vi "Create Task.vi"(8 "error in (no error)":errorcluster, 9 "Task Type":string, 10 "Task Name":string, 11 "Node in":refnum<class "Node.lvclass">) -> (0 "error out":errorcluster, 2 "Task":refnum<class "Task.lvclass">, 3 "Node out":refnum<class "Node.lvclass">)   [LabVIEW 2020, in "VolatusConfig.lvlib" / "Node.lvclass"]
uses:
  Node.lvclass
  Node.lvclass/Node.ctl
  VolatusConfigElement/VolatusConfigElement.lvclass
  VolatusConfig.lvlib
  Meta Type.ctl
  lv-cdm/CDM-Config/Config Filter/Config Lookup.lvclass
  C:/dev/lv20CE/relink/lv-volatus/VolatusConfig/VolatusConfigElement/VolatusConfigElement.lvclass
  C:/dev/lv20CE/relink/lv-volatus/VolatusConfig/Node/Node.lvclass
  Task/Task.lvclass
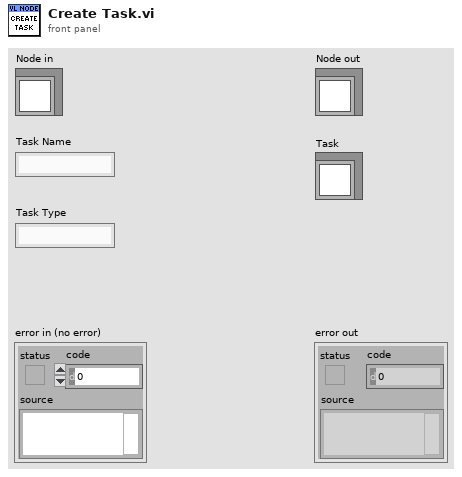
[diagram p1: front panel]
types:
  T1 = typedef "VolatusConfig.lvlib/Meta Type.ctl" = enum16{"UNKNOWN", "VL_System", "VL_Cluster", "VL_Node", "VL_Task", "VL_Group", "VL_Channel", "VL_Task_List", "VL_Scaling", "VL_Sensor", "VL_Sensor_List", "VL_Scale"}
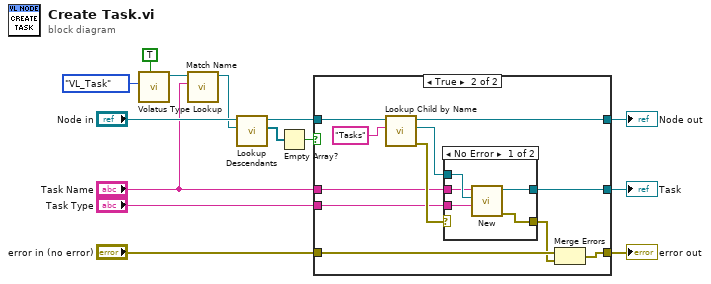
[diagram p0: block diagram]
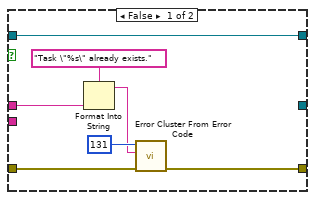
[diagram p2: hidden frame]
diagram:
  n1 = call "Volatus Type Lookup.vi"("Don't Recurse Past Match (F)"=TRUE, "Meta Type"=Meta_Type."VL_Task") -> ("Config Lookup out"=w12:refnum<class "Config Lookup.lvclass">)  [unwired: 8 in, 1 out]
  n2 = call "Match Name.vi"("Name"="Task Name", "Config Lookup (New)"=w12) -> ("Config Lookup out"=w11:refnum<class "Config Lookup.lvclass">)  [unwired: 8 in, 1 out]
  n3 = call "Lookup Descendants.vi"("Lookup"=w11, "VolatusConfigElement in"="Node in") -> ("Descendants"=w9:refnum<class "Config Element.lvclass">[], "VolatusConfigElement out"=w8:refnum<class "Node.lvclass">)  [unwired: 7 in, 1 out]
  n4 = Empty Array?(array=w9) -> (empty?=w7:bool)
  n5 = case shown="True" w7 {
    tunnel: w8 -> [w15 w32]
    tunnel: "error in (no error)" -> [w21 w26]
    tunnel: "Task Name" -> [w19 w28]
    tunnel: "Task Type" -> [_ w27]
    tunnel: [w16 w24] -> w3
    tunnel: [_ w23] -> w2
    tunnel: [w15 w22] -> w1
    frame False {
      n6 = Format Into String(format string="Task \"%s\" already exists.", w19) -> (resulting string=w17:string)  [unwired: 2 in, 1 out]
      n7 = call <vilib>:"Error Cluster From Error Code.vi"("error in (no error)"=w21, "error message (\"\")"=w17, "error code (0)"=131) -> ("error out"=w16:errorcluster)  [unwired: 6 in]
    }
    frame True {
      n8 = call "Lookup Child by Name.vi"("Child Name"="Tasks", "VolatusConfigElement in"=w32) -> ("error out"=w29:errorcluster, "Child"=w30:refnum<class "Config Element.lvclass">, "VolatusConfigElement out"=w22:refnum<class "Node.lvclass">)  [unwired: 6 in, 1 out]
      n9 = case shown="No Error" w29 {
        selector: w29 -> [_ w38]
        tunnel: w30 -> [w37 _]
        tunnel: w28 -> [w36 _]
        tunnel: [w34 w38] -> w25
        tunnel: w27 -> [w35 _]
        tunnel: [w33 _] -> w23
        frame No Error {
          n10 = call "New.vi"("Type"=w35, "Parent"=w37, "Name"=w36) -> ("error out"=w34:errorcluster, "Task out"=w33:refnum<class "Task.lvclass">)  [unwired: 7 in]
        }
        frame Error {
        }
      }
      n11 = Merge Errors(w26, w25) -> (w24:errorcluster)
    }
  }
  "error out" <- w3
  "Node out" <- w1
  "Task" <- w2
